vi "GV DO delay.vi"() -> ()   [LabVIEW 2017]
panel:
  in  "DOdelay_tick":u16
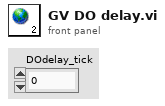
[diagram p1: front panel]
diagram:
